vi "close.vi"(8 "error in (no error)":errorcluster, 11 "DAQmx_pulse_out in":refnum<class "DAQmx_pulse_out.lvclass">) -> (0 "error out":errorcluster, 3 "DAQmx_pulse_out out":refnum<class "DAQmx_pulse_out.lvclass">)   [LabVIEW 2013, in "DAQmx_pulse_out.lvclass"]
uses:
  DAQmx_pulse_out.lvclass
  DAQmx_pulse_out.lvclass/DAQmx_pulse_out.ctl
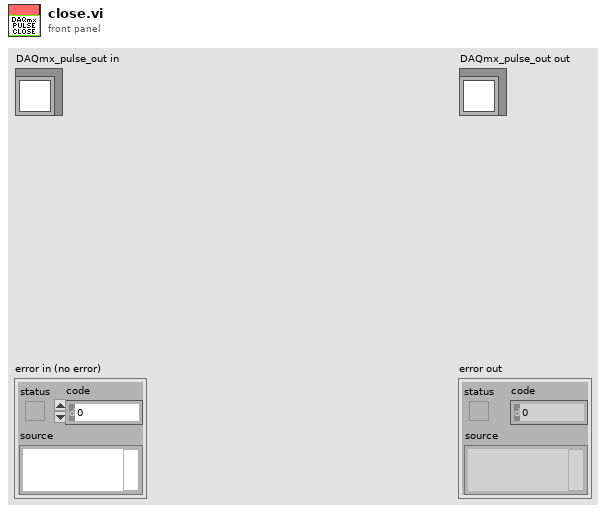
[diagram p1: front panel]
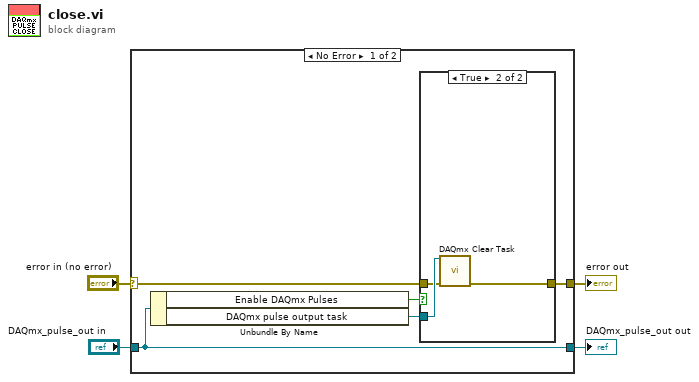
[diagram p0: block diagram]
diagram:
  n1 = case shown="No Error" "error in (no error)" {
    selector: "error in (no error)" -> [w6 w15]
    tunnel: [w5 w15] -> w3
    tunnel: [w7 w14] -> w1
    tunnel: "DAQmx_pulse_out in" -> [w7 w14]
    frame No Error {
      n2 = Unbundle By Name(w7) -> ("Enable DAQmx Pulses"=w8:bool, "DAQmx pulse output task"=w9:refnum<k21>)
      n3 = case shown="True" w8 {
        tunnel: w9 -> [_ w13]
        tunnel: w6 -> [w10 w12]
        tunnel: [w10 w11] -> w5
        frame False {
        }
        frame True {
          n4 = call <vilib>:"DAQmx Clear Task.vi"("task in"=w13, "error in"=w12) -> ("error out"=w11:errorcluster)  [unwired: 13 in]
        }
      }
    }
    frame Error {
    }
  }
  "error out" <- w3
  "DAQmx_pulse_out out" <- w1
